vi "NI VeriStand - Get Engine Rate.vi"(8 "error in (no error)":errorcluster, 11 "Item Ref in":T1 format="%.0x") -> (0 "error out":errorcluster, 2 "Rate (Hz)":dbl, 3 "Item Ref out":T1 format="%.0x")   [LabVIEW 2020, in "Custom Device API.lvlib"]
doc: "Returns the target's Primary Control Loop rate in hertz. This VI will search for the owning target of the node passed in. If you pass a target node, it will return the target's rate."
uses:
  <vilib>/NI VeriStand/Custom Device API/Custom Device API.lvlib
  <vilib>/NI VeriStand/Custom Device API/Custom Device Item Ref.ctl
  f4bbc782-2943-45fc-ab7d-3d764986fa20.vi
  <vilib>/NI VeriStand/Custom Device API/Custom Device Offline Path.vi
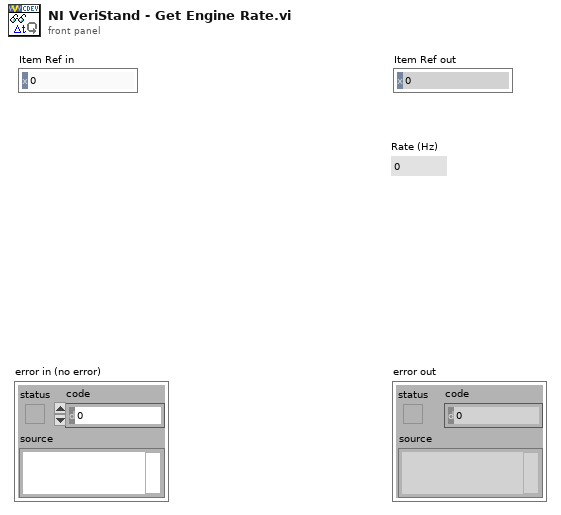
[diagram p1: front panel]
types:
  T1 = typedef "Custom Device API.lvlib/Custom Device Item Ref.ctl" = u64
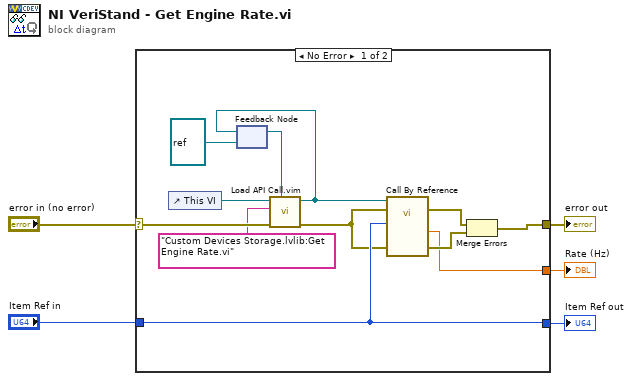
[diagram p0: block diagram]
diagram:
  n1 = case shown="No Error" "error in (no error)" {
    selector: "error in (no error)" -> [w11 w19]
    tunnel: [w16 w19] -> w5
    tunnel: "Item Ref in" -> [w14 w18]
    tunnel: [w15 _] -> w3
    tunnel: [w14 w18] -> w1
    frame No Error {
      n2 = control-ref of="This VI"() -> (w12:refnum<vi>)
      n3 = feedback #1(refnum<vi> refnum ("type specifier VI Refnum (for type only)")) -> (w13:refnum<vi>)
      n4 = call "Load API Call.vim"("VI reference in"=w13, "error in (no error)"=w11, "VI qualified name"="Custom Devices Storage.lvlib:Get Engine Rate.vi", "Caller VI ref"=w12) -> ("error out"=w7:errorcluster, "VI reference"=w10:refnum<vi>)  [unwired: 6 in]
      n5 = feedback-in #1(w10) -> ()
      n6 = call-by-ref "?"(reference=w10, error in=w7, 8:"error in (no error)"=w7, "Item Ref in"=w14) -> (error out=w6:errorcluster, 0:"error out"=w17:errorcluster, "Rate (Hz)"=w15:dbl)  [unwired: 8 in, 1 out]
      n7 = Merge Errors(w6, w17) -> (w16:errorcluster)
    }
    frame Error {
    }
  }
  "Item Ref out" <- w1
  "error out" <- w5
  "Rate (Hz)" <- w3
